vi "draw bool array.vi"(6 "Array in":bool[][](array[boolean]), 9 "min y (0)":i32, 10 "min x (0)":i32, 11 "array with duplicates removed":cluster{"x":i32, "y":i32}[](array[cluster])) -> (2 "transposed array":bool[][](array[boolean]), 3 "Array out":bool[][](array[boolean]))   [LabVIEW 2019]
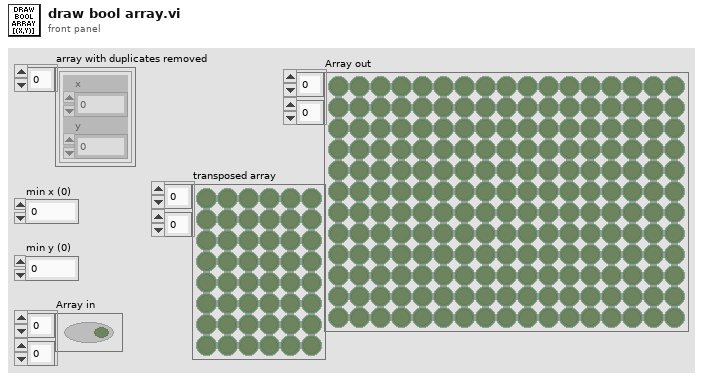
[diagram p1: front panel]
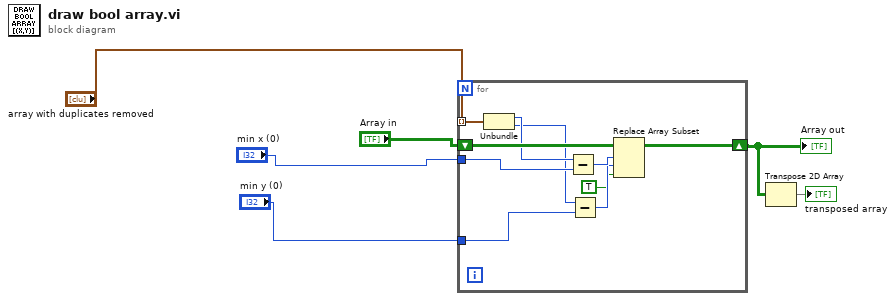
[diagram p0: block diagram]
diagram:
  n1 = for {
    tunnel: "min x (0)" -> [w15]
    tunnel: "array with duplicates removed" -> [w14] mode=indexing
    tunnel: "min y (0)" -> [w12]
    shift-right: [w7] -> w2
    shift-left: "Array in" -> [w16]
    n2 = Unbundle(w14) -> ("x"=w13:i32, "y"=w11:i32)
    n3 = Subtract(x=w13, y=w15) -> (x-y=w10:i32)
    n4 = Subtract(x=w11, y=w12) -> (x-y=w9:i32)
    n5 = Replace Array Subset(array=w16, new element=TRUE, index (row)=w10, index (col)=w9) -> (w7:bool[][])
  }
  "Array out" <- w2
  n6 = Transpose 2D Array(2D array=w2) -> (transposed array=→"transposed array":bool[][])
